vi "Get Controller Status.vi"(4 "error in (no error)":errorcluster, 7 "VISA resource name":refnum<visa-resource-name>) -> (0 "error out":errorcluster, 1 "Returned string":string, 2 "Controller Status":T1, 3 "VISA resource name out":refnum<visa-resource-name>)   [LabVIEW 2019, in "Newport ESP301.lvlib"]
doc: "Reads the controller status.\n\nRETURNS\nController Status : Cluster which returns each state of the controller\n Axis1 moving : boolean. Axis1 is moving or not\n Axis2 moving : boolean. Axis2 is moving or not\n Axis3 moving : boolean. Axis3 is moving or not\n Axis4 moving : boolean. Axis4 is moving or not\n Motor power of at least one axis : boolean. At least one motor is enable.\n Reserved : The default value is 0\n Reserved : The default value is 1\n Reserved : The default value is 0"
uses:
  Newport ESP301.lvlib
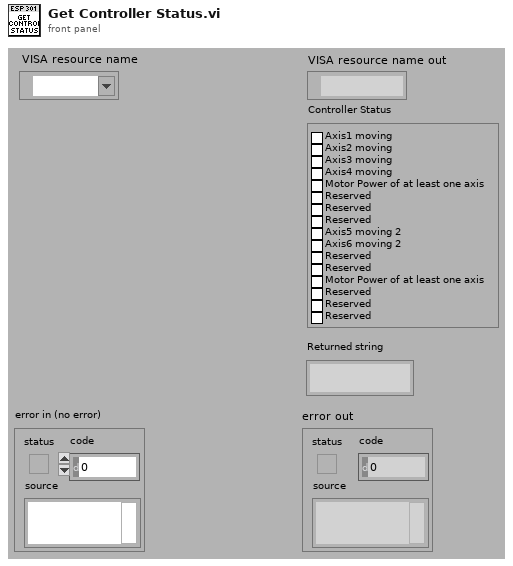
[diagram p1: front panel]
types:
  T1 = cluster{"Axis1 moving":bool, "Axis2 moving":bool, "Axis3 moving":bool, "Axis4 moving":bool, "Motor Power of at least one axis":bool, "Reserved":bool, "Reserved":bool, "Reserved":bool, "Axis5 moving 2":bool, "Axis6 moving 2":bool, "Reserved":bool, "Reserved":bool, "Motor Power of at least one axis":bool, "Reserved":bool, "Reserved":bool, "Reserved":bool}
  T2 = cluster{"Boolean array[0]":bool, "Boolean array[1]":bool, "Boolean array[2]":bool, "Boolean array[3]":bool, "Boolean array[4]":bool, "Boolean array[5]":bool, "Boolean array[6]":bool, "Boolean array[7]":bool, "Boolean array[8]":bool, "Boolean array[9]":bool, "Boolean array[10]":bool, "Boolean array[11]":bool, "Boolean array[12]":bool, "Boolean array[13]":bool, "Boolean array[14]":bool, "Boolean array[15]":bool}
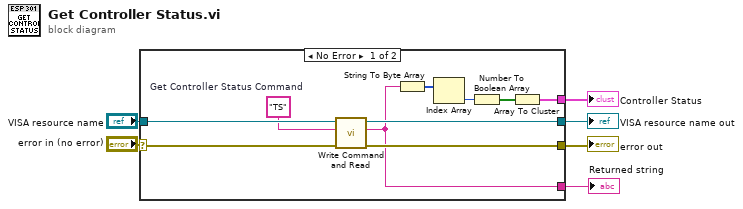
[diagram p0: block diagram]
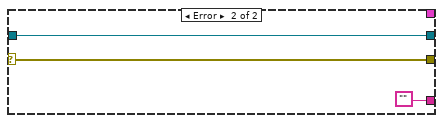
[diagram p2: hidden frame]
diagram:
  n1 = case shown="No Error" "error in (no error)" {
    selector: "error in (no error)" -> [w15 w19]
    tunnel: [w14 w19] -> w5
    tunnel: "VISA resource name" -> [w16 w18]
    tunnel: [w13 w18] -> w3
    tunnel: [w9 _] -> w2
    tunnel: [w7 ""] -> w1
    frame No Error {
      w8 = "TS"  # Get Controller Status Command
      n2 = call "Write Command and Read.vi"("error in (no error)"=w15, "Command"=w8, "VISA resource name"=w16) -> ("error out"=w14:errorcluster, "Returned string"=w7:string, "VISA resource name out"=w13:refnum<visa-resource-name>)  [unwired: 4 in]
      n3 = String To Byte Array(string=w7) -> (unsigned byte array=w12:u8[])
      n4 = Index Array(array=w12) -> (element=w11:u8)  [unwired: 1 in]
      n5 = Number To Boolean Array(number=w11) -> (Boolean array=w10:bool[])
      n6 = Array To Cluster(array=w10) -> (cluster=w9:T2)
    }
    frame Error {
    }
  }
  "error out" <- w5
  "VISA resource name out" <- w3
  "Controller Status" <- w2
  "Returned string" <- w1
